vi "Read Y.vi"(8 "error in (no error)":errorcluster, 11 "DAQmx Lockin Digitizer Driver in":refnum<class "DAQmx Lockin Digitizer Driver.lvclass">) -> (0 "error out":errorcluster, 2 "Y":dbl[](array[numeric]), 3 "DAQmx Lockin Digitizer Driver out":refnum<class "DAQmx Lockin Digitizer Driver.lvclass">)   [LabVIEW 2021, in "DAQmx Lockin Digitizer Driver.lvclass"]
uses:
  DAQmx Lockin Digitizer Driver.lvclass
  DAQmx Lockin Digitizer Driver.lvclass/DAQmx Lockin Digitizer Driver.ctl
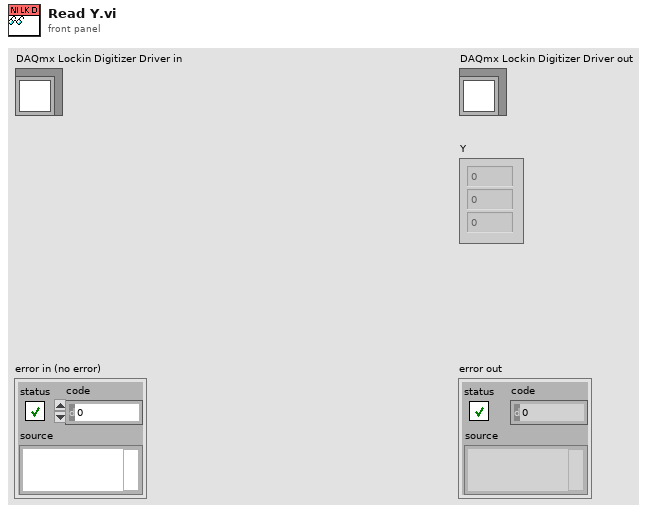
[diagram p1: front panel]
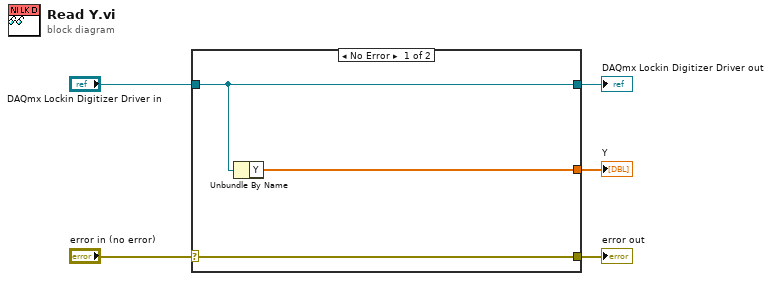
[diagram p0: block diagram]
diagram:
  n1 = case shown="No Error" "error in (no error)" {
    selector: "error in (no error)" -> [w8 w9]
    tunnel: [w8 w9] -> w4
    tunnel: [w7 w10] -> w2
    tunnel: "DAQmx Lockin Digitizer Driver in" -> [w7 w10]
    tunnel: [w6 _] -> w1
    frame No Error {
      n2 = Unbundle By Name(w7) -> ("Y"=w6:dbl[])
    }
    frame Error {
    }
  }
  "error out" <- w4
  "DAQmx Lockin Digitizer Driver out" <- w2
  "Y" <- w1
